vi "myRIO_BRig_Host_stateIdxList_timeout.vi"() -> (1 "output_min_timeout":u16=32, 3 "output_max_timeout":u16=35)   [LabVIEW 2014]
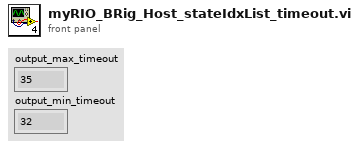
[diagram p1: front panel]
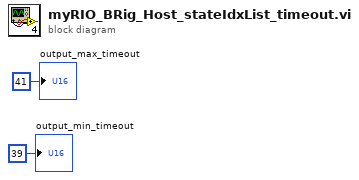
[diagram p0: block diagram]
diagram:
  "output_max_timeout" <- u16 41
  "output_min_timeout" <- u16 39
